vi "Configure SRE.vi"(8 "error in (no error)":errorcluster, 10 "value":u32 max=255 step=1, 11 "VISA resource name":refnum<visa-resource-name>) -> (0 "error out":errorcluster, 3 "VISA resource name out":refnum<visa-resource-name>)   [LabVIEW 2025]
panel:
  # "*SRE"
  # "Service Request Enable"
  # "0...255"
  # "Bit  Description\n0    Not Used\n1    Has Result\n2    Error/Event Query\n3    Not Used\n4    Message Available\n5    Standard Event\n6    Request Service\n7    Not Used"
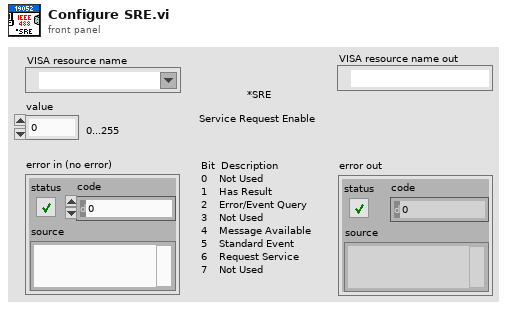
[diagram p1: front panel]
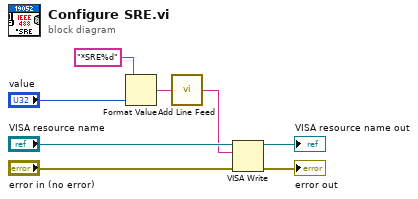
[diagram p0: block diagram]
diagram:
  n1 = Format Value(format string="*SRE%d", value (0)="value") -> (output string=w7:string)  [unwired: 1 in]
  n2 = call <instrlib>:"Add Line Feed.vi"("Command string"=w7) -> ("Concatenated string"=w1:string)  [unwired: 4 in]
  n3 = VISA Write(VISA resource name="VISA resource name", write buffer=w1, error in (no error)="error in (no error)") -> (VISA resource name out=→"VISA resource name out":refnum<visa-resource-name>, error out=→"error out":errorcluster)  [unwired: 1 out]
